vi "Gear.vi"(11 "solenoid in":T1) -> (0 "Gear time out":u32, 3 "solenoid out":T1)   [LabVIEW 2016]
uses:
  <vilib>/Rock Robotics/WPI/Solenoid/WPI_SolenoidValue.ctl
  <vilib>/Rock Robotics/WPI/Solenoid/WPI_SolenoidSetEnum.vi
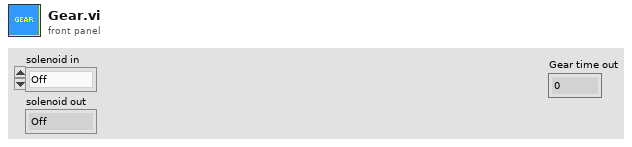
[diagram p1: front panel]
types:
  T1 = typedef "WPI_SolenoidValue.ctl" = enum16{"Off", "On", "Forward", "Reverse"}
  T2 = typedef "WPI_SolenoidDevRef.ctl" = cluster{"DevStatus":errorcluster, "Pneumatics Control Module":u8, "Forward Solenoid Channel":T3, "Reverse Solenoid Channel":T3}
  T3 = typedef "WPI_SolenoidChannel.ctl" = enum8{"Solenoid 0", "Solenoid 1", "Solenoid 2", "Solenoid 3", "Solenoid 4", "Solenoid 5", "Solenoid 6", "Solenoid 7", "Invalid"}
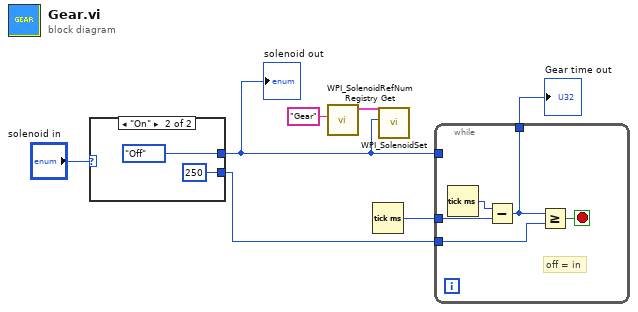
[diagram p0: block diagram]
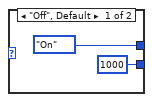
[diagram p2: hidden frame]
diagram:
  n1 = case shown="\"On\"" "solenoid in" {
    tunnel: [WPI_SolenoidValue."On" ("Value") WPI_SolenoidValue."Off" ("Value")] -> w3
    tunnel: [u32 1000 ("y") u32 250 ("y")] -> w2
    frame "Off", Default {
    }
    frame "On" {
    }
  }
  "solenoid out" <- w3
  n2 = call <vilib>:"WPI_SolenoidRefNum Registry Get.vi"("refnum name"="Gear") -> ("SolenoidDevRef"=w6:T2)  [unwired: 9 in, 1 out]
  n3 = Tick Count (ms)() -> (millisecond timer value=w7:u32)
  n4 = call-poly <vilib>:"WPI_SolenoidSet.vi"("Value"=w3, "SolenoidDevRef"=w6) -> ()  [unwired: 8 in, 2 out]
  n5 = while {
    tunnel: w7 -> [w15]
    tunnel: w3 -> [_]
    tunnel: w2 -> [w13]
    tunnel: [w12] -> w1
    stop <- w14 stop-if-true
    # "off = in"
    n6 = Tick Count (ms)() -> (millisecond timer value=w16:u32)
    n7 = Subtract(x=w16, y=w15) -> (x-y=w12:u32)
    n8 = Greater Or Equal?(x=w12, y=w13) -> (x >= y?=w14:bool)
  }
  "Gear time out" <- w1
